vi "Set Parent(MDI).vi"(8 "Error In":errorcluster, 9 "Panel":refnum<k24>, 10 "Number of socket":i32, 11 "Test Executive Manage in":refnum<class "Test Executive Manage.lvclass">) -> (0 "Error Out":errorcluster, 1 "UUT Result":map{i32, refnum<user-event>}(c390), 2 "exit":refnum<user-event>[](array[refnum]), 3 "Test Executive Manage out":refnum<class "Test Executive Manage.lvclass">, 5 "UserMessage":map{i32, refnum<user-event>}(c390))   [LabVIEW 2025, in "Test Unit.lvlib"]
uses:
  Test Unit.lvlib
  System.Windows.Forms
  <vilib>/Test Bench Framework/Test Executive.lvlibp/TestEngine/Test Executive Manage/Test Executive Manage.lvclass
  UUT Result.ctl
  <vilib>/Test Bench Framework/Test Executive.lvlibp/TestEngine/TestEngine/TestEngine/Typedefs/Report General.ctl
  Full User Interface/Send User Message Argument--cluster.ctl
  <vilib>/Test Bench Framework/Test Executive(API).lvlib
  <vilib>/Test Bench Framework/Test Executive.lvlibp/TestEngine/TestEngine/TestEngine/Test Engine.lvclass
  Full User Interface/Full User Interface.lvlib
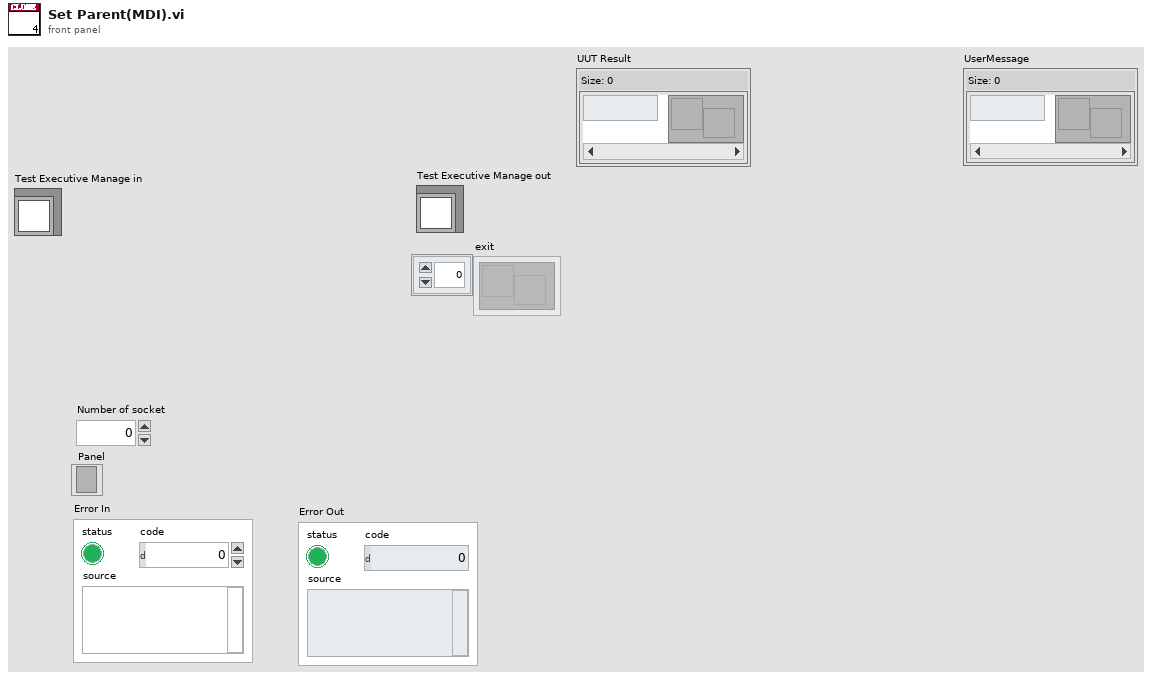
[diagram p1: front panel]
types:
  T1 = cluster{"UUT State":refnum<vi>, "Cycle Time":refnum<vi>, "SerialNumber":refnum<vi>, "Tree":refnum<vi>, "This VI":refnum<vi>}
  T2 = cluster{"UUT State":refnum<vi>, "Cycle Time":refnum<vi>, "SerialNumber":refnum<vi>}
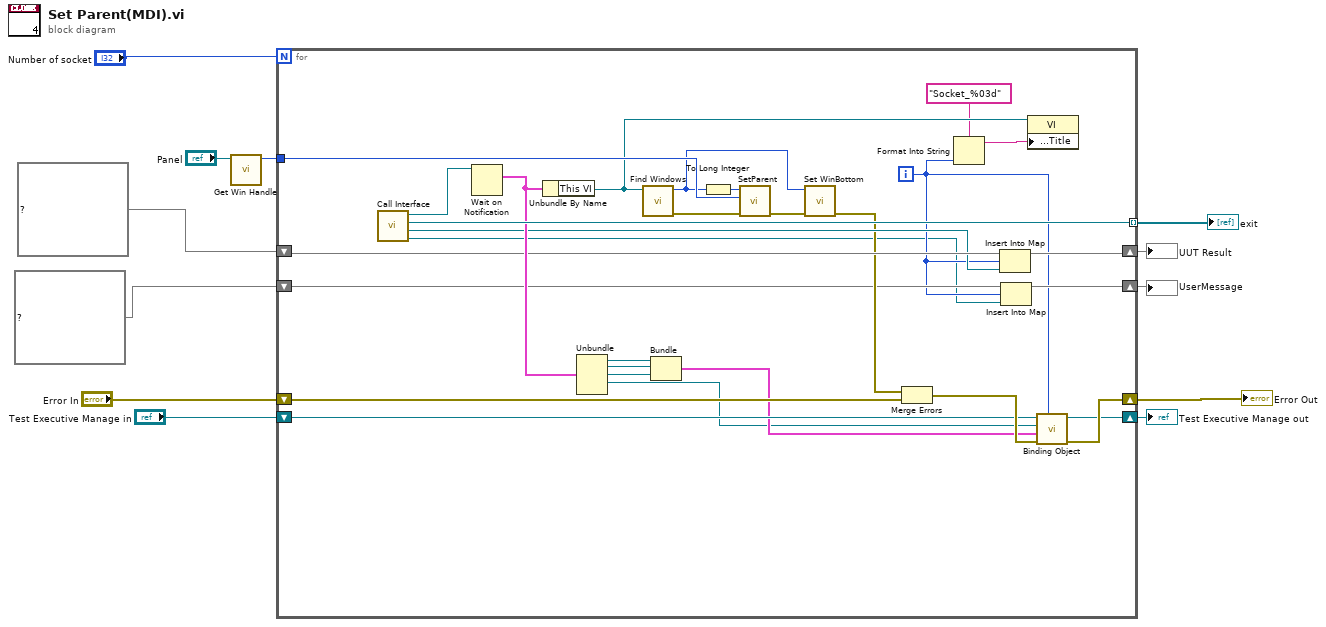
[diagram p0: block diagram]
diagram:
  n1 = call "Get Win Handle.vi"(".NET Refnum in"="Panel") -> ("ToInt32"=w6:i32)  [unwired: 7 in, 3 out]
  n2 = for {
    N: "Number of socket" -> [_]
    tunnel: [w41] -> w11 mode=indexing
    shift-right: [w32] -> w5
    shift-left: "Error In" -> [w40]
    shift-right: [w31] -> w8
    shift-left: "Test Executive Manage in" -> [w30]
    tunnel: w6 -> [w27]
    shift-right: [w22] -> w3
    shift-left: map{i32, refnum<user-event>} {} ("map") -> [w23]
    shift-right: [w15] -> w1
    shift-left: map{i32, refnum<user-event>} {} ("map") -> [w16]
    i -> [w14]
    n3 = call "Call Interface.vi"() -> ("UserMessage"=w13:refnum<user-event>, "UUT Result"=w21:refnum<user-event>, "exit"=w41:refnum<user-event>, "ref"=w39:refnum<notifier>)  [unwired: 8 in]
    n4 = Wait on Notification(notifier=w39) -> (notification=w37:T1)  [unwired: 3 in, 3 out]
    n5 = Unbundle By Name(w37) -> ("This VI"=w26:refnum<vi>)
    n6 = Unbundle(w37) -> ("UUT State"=w36:refnum<vi>, "Cycle Time"=w35:refnum<vi>, "SerialNumber"=w34:refnum<vi>, "Tree"=w28:refnum<vi>)  [unwired: 1 out]
    n7 = call "Find Windows.vi"("VI reference"=w26) -> ("error out"=w38:errorcluster, "hWnd"=w17:u32)  [unwired: 9 in]
    n8 = Bundle("UUT State"=w36, "Cycle Time"=w35, "SerialNumber"=w34) -> (w29:T2)  [unwired: 1 in]
    n9 = To Long Integer(number=w17) -> (32bit integer=w19:i32)
    n10 = call "SetParent.vi"("error in (no error)"=w38, "hWndNewParent"=w27, "hWndChild"=w19) -> ("error out"=w20:errorcluster)  [unwired: 7 in, 1 out]
    n11 = call "Set WinBottom.vi"("error in (no error)"=w20, "hWnd"=w17) -> ("error out"=w18:errorcluster)  [unwired: 9 in]
    n12 = Merge Errors(w18, w40) -> (w33:errorcluster)
    n13 = Format Into String(format string="Socket_%03d", w14) -> (resulting string=w24:string)  [unwired: 2 in, 1 out]
    n14 = Insert Into Map(map in=w23, key=w14, value=w21) -> (map out=w22:map{i32, refnum<user-event>})  [unwired: 2 out]
    n15 = Insert Into Map(map in=w16, key=w14, value=w13) -> (map out=w15:map{i32, refnum<user-event>})  [unwired: 2 out]
    n16 = property class="VI"(reference=w26, "Front Panel.Title"=w24) -> ()  [unwired: 1 in, 2 out]
    n17 = call <vilib>:"Binding Object.vi"("Socket"=w14, "error in (no error)"=w33, "Result"=w29, "Items List Reference"=w28, "Test Executive Manage in"=w30) -> ("error out"=w32:errorcluster, "Test Executive Manage out"=w31:refnum<class "Test Executive Manage.lvclass">)  [unwired: 5 in]
  }
  "Error Out" <- w5
  "exit" <- w11
  "Test Executive Manage out" <- w8
  "UUT Result" <- w3
  "UserMessage" <- w1
